vi "Initialize PEM.vi"(8 "error in (no error)":errorcluster, 11 "VISA resource name":refnum<visa-resource-name>="COM4") -> (0 "error out":errorcluster, 3 "VISA resource name out":refnum<visa-resource-name>)   [LabVIEW 2023]
panel:
  out "Echo output":string
  # "Should be a question Mark"
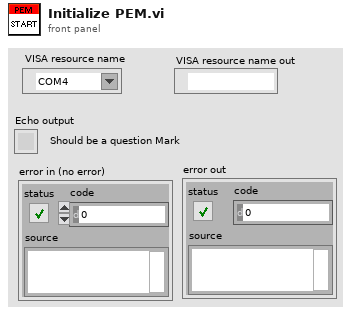
[diagram p1: front panel]
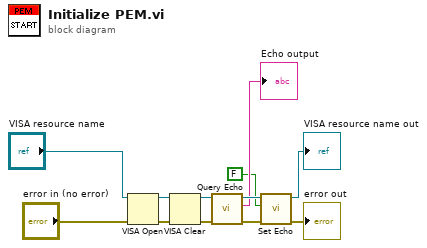
[diagram p0: block diagram]
diagram:
  n1 = VISA Open(error in (no error)="error in (no error)", VISA resource name="VISA resource name") -> (VISA resource name=w9:refnum<visa-resource-name>, error out=w10:errorcluster)  [unwired: 3 in]
  n2 = VISA Clear(VISA resource name=w9, error in (no error)=w10) -> (VISA resource name out=w7:refnum<visa-resource-name>, error out=w8:errorcluster)
  n3 = call "Query Echo.vi"("error in (no error)"=w8, "VISA resource name"=w7) -> ("error out"=w5:errorcluster, "Echo output"=→"Echo output":string, "VISA resource name out"=w6:refnum<visa-resource-name>)  [unwired: 7 in]
  n4 = call "Set Echo.vi"("error in (no error)"=w5, "Echo"=FALSE, "VISA resource name"=w6) -> ("error out"=→"error out":errorcluster, "VISA resource name out"=→"VISA resource name out":refnum<visa-resource-name>)  [unwired: 6 in, 1 out]
